vi "XML_TestMessage.vi"(0 "Unit Timestamp":string, 1 "SerialNumber":string, 2 "StatusCode":string, 3 "DateTimeStart":string, 4 "DateTimeEnd":string, 5 "error in (no error)":errorcluster caption="错误输入（无错误）") -> (14 "连接的字符串":string, 19 "error out":errorcluster caption="错误输出")   [LabVIEW 2018]
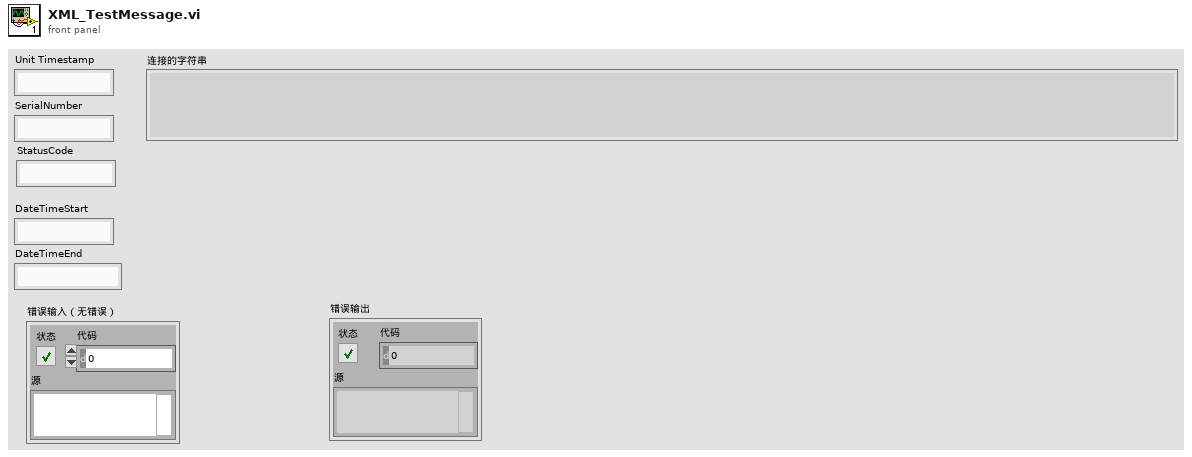
[diagram p1: front panel]
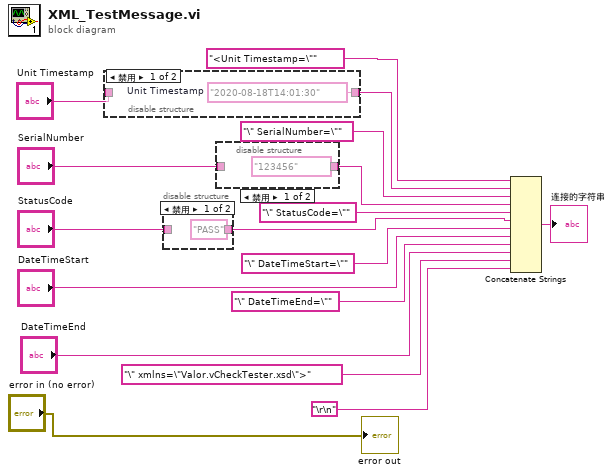
[diagram p0: block diagram]
diagram:
  n1 = disable-structure shown="禁用" {
    disable-tunnel: [w18 w19] -> w14
    disable-tunnel: "Unit Timestamp" -> [_ w19]
    frame Disabled {
      w18 = "2020-08-18T14:01:30"  # Unit Timestamp
    }
    frame Enabled {
    }
  }
  n2 = disable-structure shown="禁用" {
    disable-tunnel: ["PASS" w21] -> w17
    disable-tunnel: "StatusCode" -> [_ w21]
    frame Disabled {
    }
    frame Enabled {
    }
  }
  n3 = disable-structure shown="禁用" {
    disable-tunnel: ["123456" w23] -> w16
    disable-tunnel: "SerialNumber" -> [_ w23]
    frame Disabled {
    }
    frame Enabled {
    }
  }
  n4 = Concatenate Strings("<Unit Timestamp=\"", w14, "\" SerialNumber=\"", w16, "\" StatusCode=\"", w17, "\" DateTimeStart=\"", "DateTimeStart", "\" DateTimeEnd=\"", "DateTimeEnd", "\" xmlns=\"Valor.vCheckTester.xsd\">", "\r\n") -> (→"连接的字符串":string)
  "error out" <- "error in (no error)"
